vi "Init.vi"(7 "Is Sync":bool) -> (3 "Setup Msg out":refnum<class "Setup Msg.lvclass">)   [LabVIEW 2021, in "jettl.lvlib" / "Setup Msg.lvlib" / "Setup Msg.lvclass"]
uses:
  Setup Msg.lvclass
  Setup Msg.lvclass/Setup Msg.ctl
  Sender/Sender.lvlib
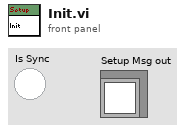
[diagram p1: front panel]
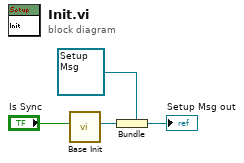
[diagram p0: block diagram]
diagram:
  n1 = call "Base Init.vi"("Is Sync"="Is Sync") -> ("Sender"=w2:refnum<class "Sender.lvclass">)  [unwired: 10 in]
  n2 = Bundle "Bundle"(cluster=refnum<class "Setup Msg.lvclass"> refnum ("Setup Msg out"), w2) -> (→"Setup Msg out":refnum<class "Setup Msg.lvclass">)
